vi "calc_movement_time_TEST.vi"() -> ()   [LabVIEW 2013]
uses:
  MCode_LV_86/Set Parameter.ctl
panel:
  in  "steps":i32
  out "MoveF":bool
  in  "Echo Mode":i32
  in  "Loop Stop":bool
  out "error out":errorcluster={"status"=FALSE, "code"=1073676294, "source"="VISA Read in write_read.vi"}
  out "VISA ressource out":refnum<visa-resource-name>
  in  "error in (no error)":errorcluster
  in  "VISA resource name":refnum<visa-resource-name>
  in  "Motor":u16(ring) items=["none", "1", "2", "3", "4", "all"]
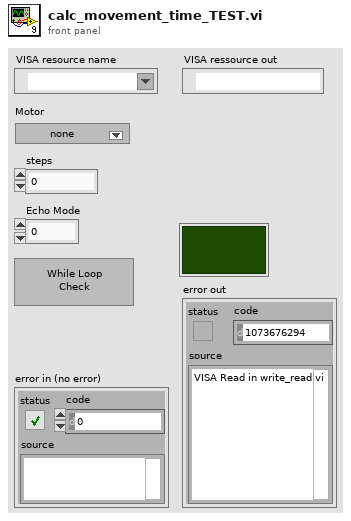
[diagram p1: front panel]
types:
  T1 = typedef "Set Parameter.ctl" = enum16{"Acceleration (A)", "Baud Rate (BD)", "Counter 1 (C1)", "Counter 2 (C2)", "Control C Software Reset (CE)", "Check Sum Enable (CK)", "Clock Mode (CM)", "Clock Mode Ratio (CR)", "Clock Mode Out Step Width (CW)", "Deceleration (D)", "Digital Filtering, Input 1 (D1)", "Digital Filtering, Input 2 (D2)", "Digital Filtering, Input 3 (D3)", "Digital Filtering, Input 4 (D4)", "Digital Filtering, Input 5 (D5)", "Digital Filtering, Input 9 (D9)", "Digital Filtering, Input 10 (D10)", "Digital Filtering, Input 11 (D11)", "Digital Filtering, Input 12 (D12)", "Deadband (DB)", "Decrement Variable (DC)", "Enable/Disable Drive (DE)", "Device Name (DN)", "End Program Execution (E)", "Encoder Function Enable (EE)", "Encoder Lines (EL)", "Echo Mode (EM)", "Error Value (ER)", "Escape (ES)", "Execute Program at Address (EX)", "Firmware Version (VR)", "Hold (H)", "Hold Current (HC)", "Hold Current Delay Time (HI)", "Home to Encoder Index (HM)", "Home to Home Switch (HT)", "Increment Variable (IC)", "Initialize Parameters to NVM (IP)", "Input into Variable (IV)", "Jog Enable (JE)", "Limit Stop Mode (LM)", "Move Absolute (MA)", "Move Relative (MR)", "MicroStepping Select (MS)", "Motor Settling Delay Time (MT)", "Moving [Flag] (MV)", "Output 1 (O1)", "Output 2 (O2)", "Output 3 (O3)", "Output 4 (O4)", "Output 9 (O9)", "Output 10 (O10)", "Output 11 (O11)", "Output 12 (O12)", "Output High Byte (9-12) (OH)", "Output Low Byte (1-4) (OL)", "Output Total (1-4 and 9-12) (OT)", "Position (P)", "Position Maintenance (PM)", "Party Mode (PY)", "Register 1 (R1)", "Register 2 (R2)", "Register 3 (R3)", "Register 4 (R4)", "Reset Error(\\03)", "Run Current (RC)", "Stall Factor (SF)", "Slew (SL)", "Stall Mode Set (SM)", "Upgrade Firmware (UG)", "Velocity Initial (VI)", "Velocity Maximum (VM)"}
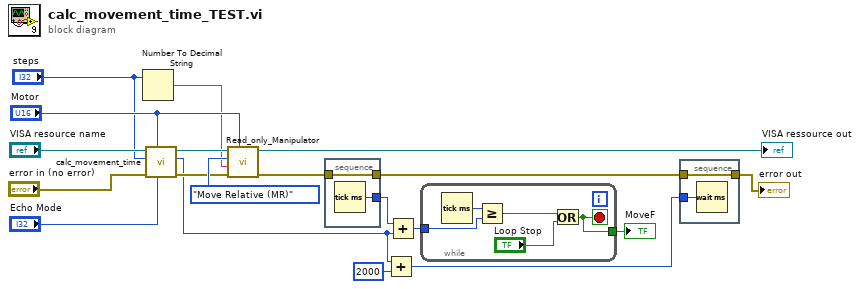
[diagram p0: block diagram]
diagram:
  n1 = Number To Decimal String(number="steps") -> (decimal integer string=w1:string)  [unwired: 1 in]
  n2 = call "calc_movement_time.vi"("Echo Mode"="Echo Mode", "Motor"="Motor", "error in (no error)"="error in (no error)", "steps"="steps", "VISA ressource in"="VISA resource name") -> ("error out"=w12:errorcluster, "move time (ms)"=w9:u32, "VISA ressource out"=w13:refnum<visa-resource-name>)  [unwired: 4 in]
  n3 = call "Read_only_Manipulator.vi"("Motor"="Motor", "error in (no error)"=w12, "Value"=w1, "Command"=Set_Parameter."Move Relative (MR)", "VISA resource name"=w13) -> ("error out"=w17:errorcluster, "VISA ressource out"=→"VISA ressource out":refnum<visa-resource-name>)  [unwired: 3 in, 2 out]
  n4 = stacked-sequence {
    tunnel: w17 -> [w21]
    tunnel: [w21] -> w6
    tunnel: [w20] -> w8
    frame #0 {
      n5 = Tick Count (ms)() -> (millisecond timer value=w20:u32)
    }
  }
  n6 = Add(x=w9, y=u32 2000) -> (x+y=w4:u32)
  n7 = Add(x=w8, y=w9) -> (x+y=w7:u32)
  n8 = while {
    tunnel: w7 -> [w25]
    tunnel: [w23] -> w3
    stop <- w23 stop-if-true
    n9 = Tick Count (ms)() -> (millisecond timer value=w26:u32)
    n10 = Greater Or Equal?(x=w26, y=w25) -> (x >= y?=w24:bool)
    n11 = Or(x=w24, y="Loop Stop") -> (x .or. y?=w23:bool)
  }
  "MoveF" <- w3
  n12 = stacked-sequence {
    tunnel: w6 -> [w28]
    tunnel: [w28] -> w5
    tunnel: w4 -> [w27]
    frame #0 {
      n13 = Wait (ms)(milliseconds to wait=w27) -> ()  [unwired: 1 out]
    }
  }
  "error out" <- w5
